vi "PropertyObject Ref.vi"(8 "error in (no error)":errorcluster, 11 "PropertyObject in":refnum<class "PropertyObject.lvclass">) -> (0 "error out":errorcluster, 2 "PropertyObject":refnum<k7>, 3 "PropertyObject out":refnum<class "PropertyObject.lvclass">)   [LabVIEW 2020, in "TSnax.lvlib" / "PropertyObject.lvclass"]
uses:
  PropertyObject.lvclass
  PropertyObject.lvclass/PropertyObject.ctl
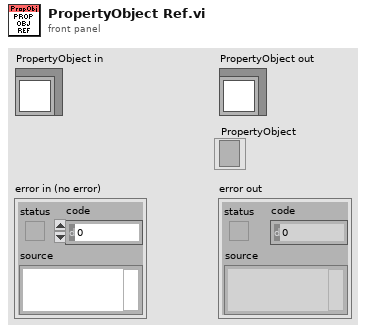
[diagram p1: front panel]
types:
  T1 = typedef "TSnax.lvlib/PropertyObject.lvclass/Ref Data.ctl" = cluster{"PropertyObject":refnum<k7>}
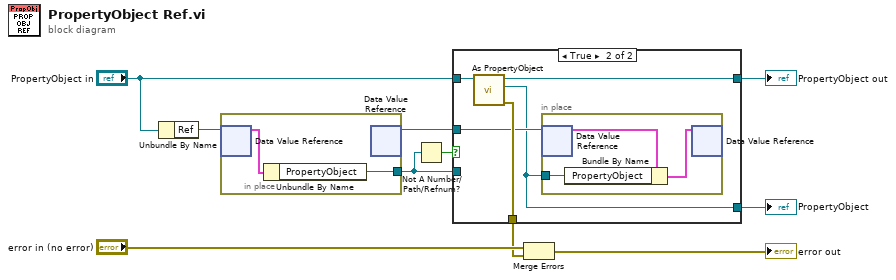
[diagram p0: block diagram]
diagram:
  n1 = Unbundle By Name("PropertyObject in") -> ("Ref"=w4:refnum<data-value>)
  n2 = in-place {
    in-place-border: [w11] -> w2
    n3 = in-place-dvr #1(w4) -> (w12:T1)  [unwired: 1 out]
    n4 = Unbundle By Name(w12) -> ("PropertyObject"=w11:refnum<k7>)
    n5 = in-place-dvr #1() -> (w1:refnum<data-value>)  [unwired: 1 in, 1 out]
  }
  n6 = Not A Number/Path/Refnum?(number/path/refnum=w2) -> (NaN/Path/Refnum?=w9:bool)
  n7 = case shown="True" w9 {
    tunnel: w2 -> [w13 _]
    tunnel: "PropertyObject in" -> [w14 w19]
    tunnel: [w14 w15] -> w8
    tunnel: [_ w18] -> w6
    tunnel: [w13 w16] -> w5
    tunnel: w1 -> [_ w17]
    frame False {
    }
    frame True {
      n8 = call-dynamic "As PropertyObject.vi"("PropertyObject in"=w19) -> ("error out"=w18:errorcluster, "PropertyObject"=w16:refnum<k7>, "PropertyObject out"=w15:refnum<class "PropertyObject.lvclass">)  [unwired: 8 in]
      n9 = in-place {
        in-place-border: w16 -> [w20]
        n10 = in-place-dvr #2(w17) -> (w22:T1)  [unwired: 1 out]
        n11 = Bundle By Name(cluster=w22, "PropertyObject"=w20) -> (w21:T1)
        n12 = in-place-dvr #2(w21) -> ()  [unwired: 2 out]
      }
    }
  }
  "PropertyObject out" <- w8
  "PropertyObject" <- w5
  n13 = Merge Errors("error in (no error)", w6) -> (→"error out":errorcluster)
